vi "dialog.change.string.vi"(11 "Issue Name":string) -> (2 "apply?":bool, 3 "issue name out":string)   [LabVIEW 2024]
panel:
  in  "Confirm":bool
  in  "Cancel":bool
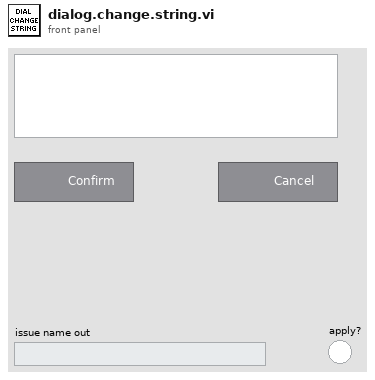
[diagram p1: front panel]
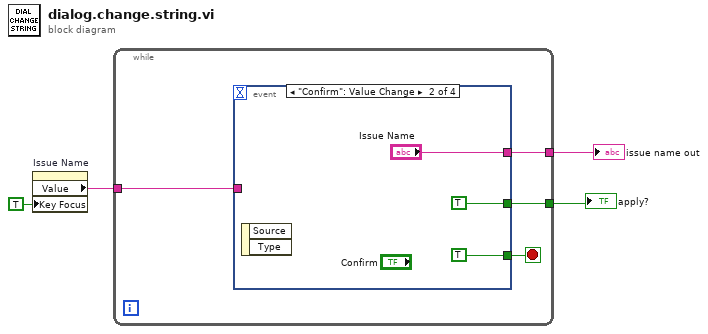
[diagram p0: block diagram]
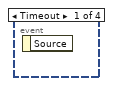
[diagram p2: hidden frame]
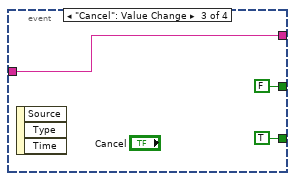
[diagram p3: hidden frame]
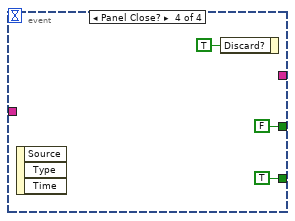
[diagram p4: hidden frame]
diagram:
  n1 = property on="Issue Name" class="Str"("Key Focus"=TRUE) -> ("Value"=w4:string)  [unwired: 2 in, 2 out]
  n2 = while {
    tunnel: w4 -> [w8]
    tunnel: [w7] -> w3
    tunnel: [w6] -> w2
    stop <- w5 stop-if-true
    n3 = event shown="[1] \"Confirm\": Value Change" {
      selector: _ -> [_ _ _ _]
      dyn-events: _ -> [_ _ _ _]
      timeout: _ -> [_ _ _ _]
      tunnel: w8 -> [_ _ w13 _]
      tunnel: [_ "Issue Name" w13 _] -> w7
      tunnel: [_ TRUE FALSE FALSE] -> w6
      tunnel: [_ TRUE TRUE TRUE] -> w5
      event Timeout {
        n4 = event-data() -> ()  [unwired: 1 in, 1 out]
      }
      event "Confirm": Value Change {
        n5 = event-data() -> ()  [unwired: 1 in, 2 out]
      }
      event "Cancel": Value Change {
        n6 = event-data() -> ()  [unwired: 1 in, 3 out]
      }
      event Panel Close? {
        n7 = event-data() -> ()  [unwired: 1 in, 3 out]
        n8 = event-data("Discard?"=TRUE) -> ()  [unwired: 1 in, 1 out]
      }
    }
  }
  "issue name out" <- w3
  "apply?" <- w2
